vi "Curtin1_Lists.vi"(10 "Old Files":T1[](array[typedef])) -> (2 "New Files":T1[](array[typedef]))   [LabVIEW 2022 SP3]
uses:
  Curtin1_Label.ctl
panel:
  in  "Append":bool
  in  "description":string
  in  "Replace":bool
  in  "Add List":bool
  in  "Save As":bool
  in  "Save":bool
  in  "delete":bool
  in  "Export":bool
  in  "Remove":bool
  in  "List Files":i32[](listbox)
  in  "Add":bool
  in  "Possible Lists":i32(listbox)
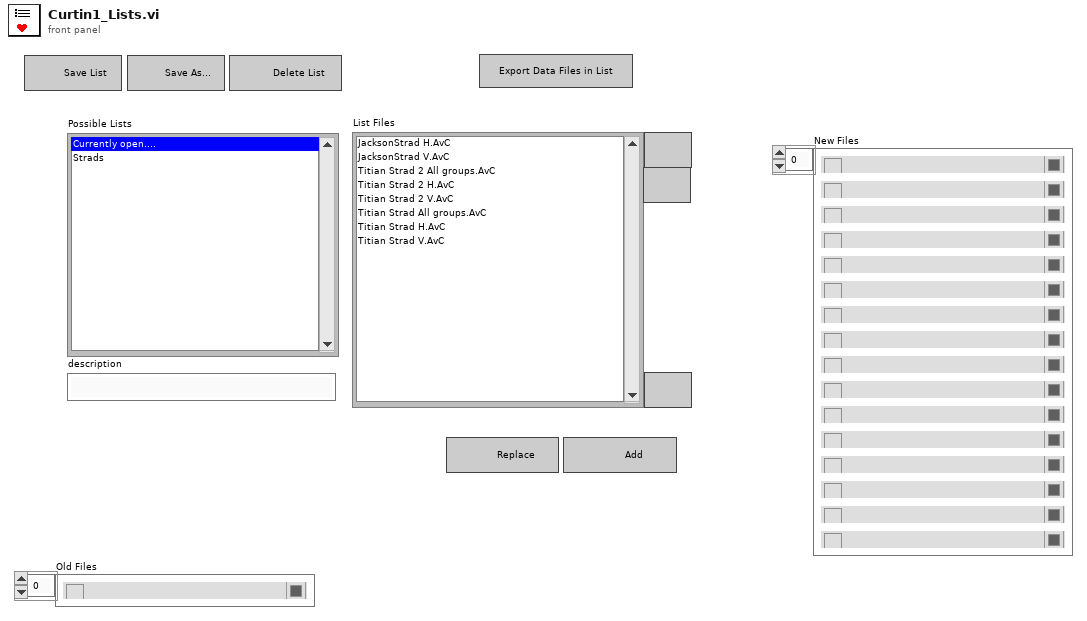
[diagram p1: front panel]
types:
  T1 = typedef "Curtin1_Label.ctl" = cluster{"Show?":bool, "Name":string, "Color":u32, "Path":path, "Show Notes":bool}
  T2 = enum8{"Enabled", "Disabled", "Disabled and Grayed Out"}
  T3 = enum32{"Invalid", "Default", "Floating", "Floating/Auto-Hide", "Modal"}
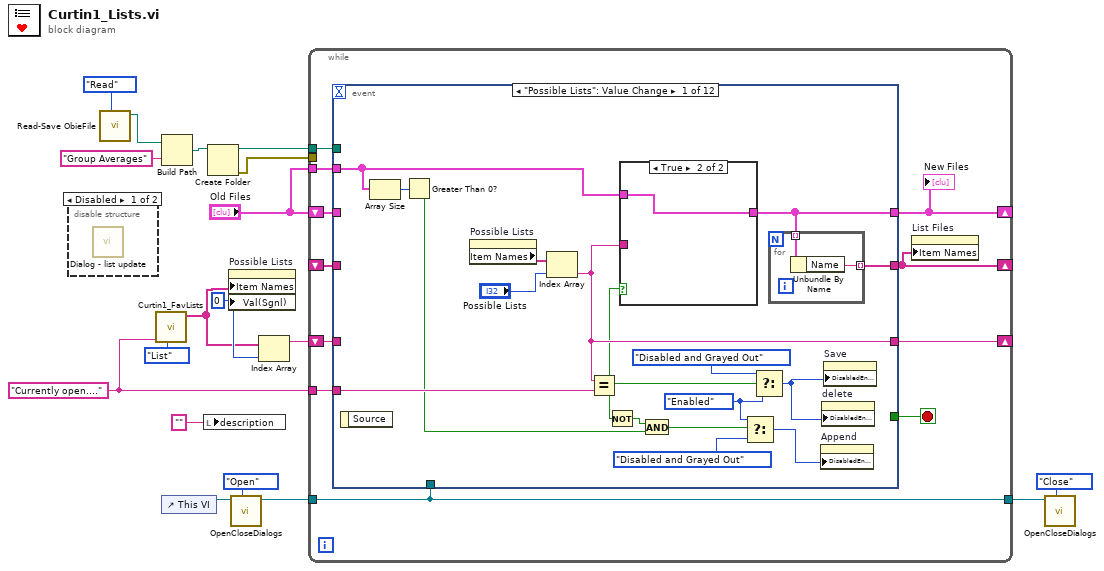
[diagram p0: block diagram]
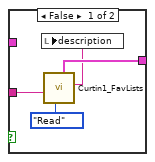
[diagram p3: hidden frame]
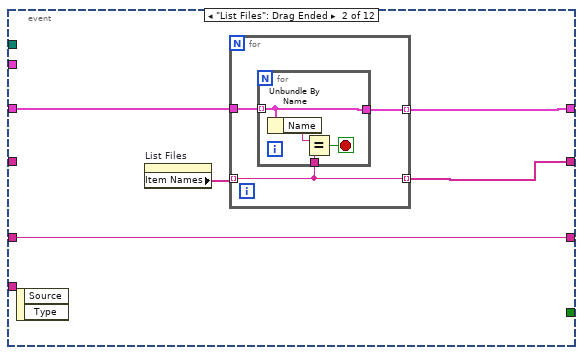
[diagram p4: hidden frame]
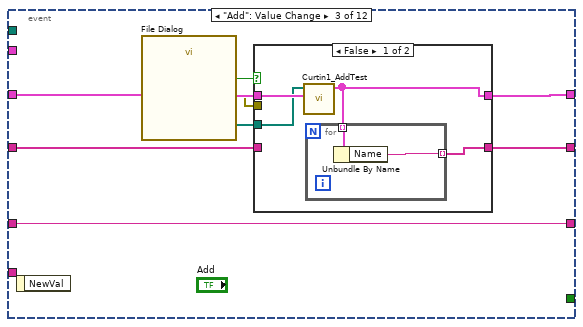
[diagram p5: hidden frame]
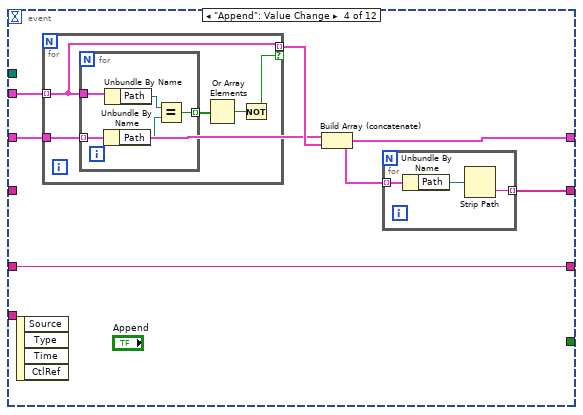
[diagram p7: hidden frame]
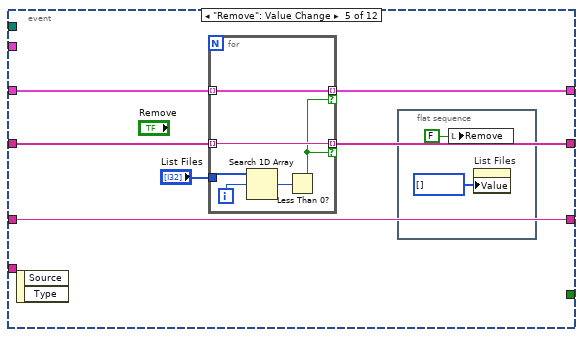
[diagram p8: hidden frame]
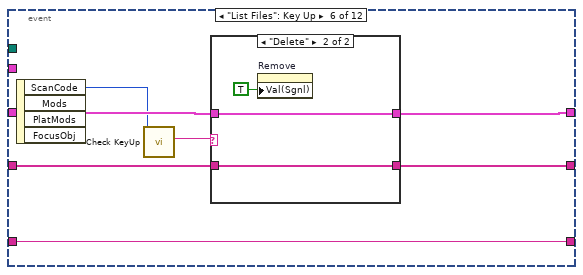
[diagram p9: hidden frame]
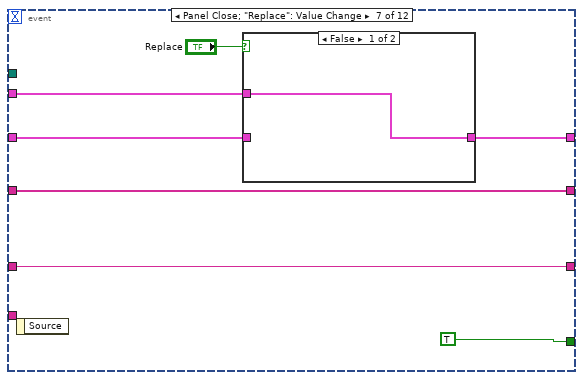
[diagram p11: hidden frame]
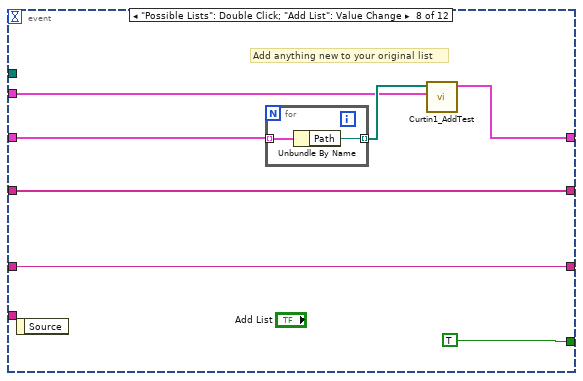
[diagram p13: hidden frame]
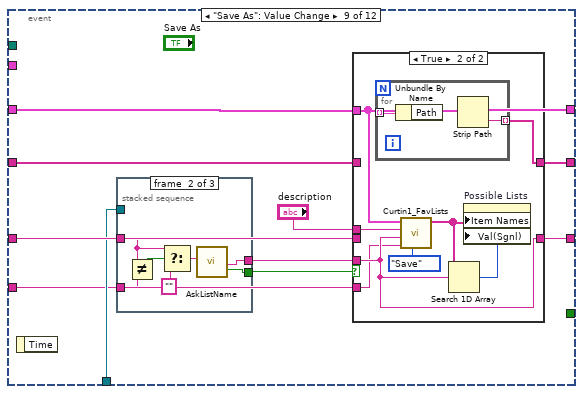
[diagram p14: hidden frame]
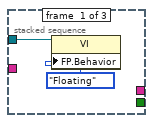
[diagram p15: hidden frame]
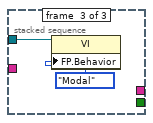
[diagram p16: hidden frame]
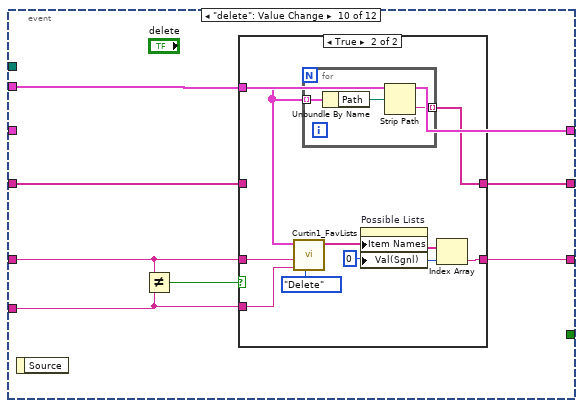
[diagram p18: hidden frame]
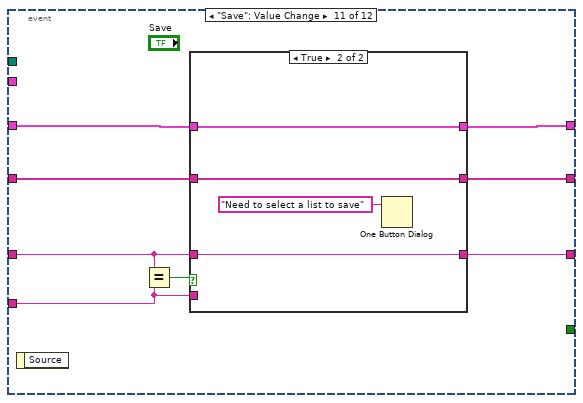
[diagram p20: hidden frame]
diagram:
  w14 = "Currently open...." ("List Name")
  w18 = u16 0 ("Value (Signaling)")
  n1 = disable-structure shown="Disabled" {
    frame Disabled {
      n2 = call "Dialog - list update.vi"() -> ()  [unwired: 10 in, 2 out]
    }
    frame Enabled {
    }
  }
  n3 = call "Read-Save ObieFile.vi"("Task"=enum16{"Save", "Read"}."Read") -> ("DataPath Out"=w12:path)  [unwired: 8 in, 2 out]
  n4 = call "Curtin1_FavLists.vi"("Task"=enum16{"Save", "Read", "List"}."List", "Default"=w14) -> ("Lists"=w1:string[])  [unwired: 6 in, 3 out]
  n5 = Build Path(base path=w12, name or relative path="Group Averages") -> (appended path=w10:path)
  n6 = control-ref of="This VI"() -> (w6:refnum<vi>)
  n7 = local write "description"("" ("description")) -> ()
  n8 = Create Folder(path (use dialog)=w10) -> (created path=w9:path, error out=w8:errorcluster)  [unwired: 2 in, 1 out]
  n9 = property on="Possible Lists" class="LstBox (strict)"("Item Names"=w1, "Val(Sgnl)"=w18) -> ()  [unwired: 2 in, 2 out]
  n10 = call "OpenCloseDialogs.vi"("Task"=enum16{"Open", "Close"}."Open", "VI in"=w6) -> ("VI out"=w3:refnum<vi>)  [unwired: 8 in, 1 out]
  n11 = Index Array(array=w1, index=w18) -> (element=w17:string)
  n12 = while {
    shift-right: [w28] -> _
    shift-left: _ -> [w29]
    shift-right: [w26] -> _
    shift-left: w17 -> [w25]
    shift-right: [w20] -> _
    shift-left: "Old Files" -> [w24]
    tunnel: "Old Files" -> [w23]
    tunnel: w14 -> [w22]
    tunnel: w9 -> [w21]
    tunnel: w8 -> [_]
    tunnel: [w19] -> w4
    tunnel: w3 -> [w19]
    stop <- w27 stop-if-true
    n13 = event shown="[0] \"Possible Lists\": Value Change" {
      selector: _ -> [_ _ _ _ _ _ _ _ _ _ _ _]
      dyn-events: _ -> [_ _ _ _ _ _ _ _ _ _ _ _]
      timeout: _ -> [_ _ _ _ _ _ _ _ _ _ _ _]
      tunnel: w29 -> [_ _ w73 _ w101 w121 w132 w142 w153 w179 w200 w223]
      tunnel: [w44 w55 w72 w82 w102 w120 w132 w142 w154 w184 w201 w223] -> w28
      tunnel: [_ _ _ _ _ _ TRUE ("OK Button") TRUE ("OK Button") _ _ _ _] -> w27
      tunnel: [w41 w54 w69 w87 w106 w119 w131 w141 w152 w182 w205 w219] -> w26
      tunnel: w25 -> [_ w54 w69 w87 w106 w119 w131 w141 w150 w181 w199 w219]
      tunnel: w24 -> [_ w58 w71 w84 w103 w118 w128 w138 w151 _ w202 w222]
      tunnel: [w43 w57 w70 w83 w104 w117 w129 w137 w151 w183 w203 w222] -> w20
      tunnel: w23 -> [w38 _ _ w86 _ _ w127 w139 _ w183 _ _]
      tunnel: w22 -> [w42 _ _ _ _ _ _ _ w145 w180 w204 _]
      tunnel: w21 -> [_ _ _ _ _ _ _ _ _ _ _ _]
      tunnel: w19 -> [_ _ _ _ _ _ _ _ w147 _ _ _]
      event "Possible Lists": Value Change {
        w32 = T2."Enabled" ("Disabled")
        n14 = event-data() -> ()  [unwired: 1 in, 1 out]
        n15 = Array Size(array=w38) -> (size(s)=w37:i32)
        n16 = Greater Than 0?(x=w37) -> (x > 0?=w34:bool)
        n17 = property on="Possible Lists" class="LstBox (strict)"() -> ("Item Names"=w46:string[])  [unwired: 2 in, 2 out]
        n18 = Index Array(array=w46, index="Possible Lists") -> (element=w41:string)
        n19 = Equal?(x=w41, y=w42) -> (x = y?=w36:bool)
        n20 = Not(x=w36) -> (.not. x?=w35:bool)
        n21 = case shown="True" w36 {
          tunnel: w41 -> [w50 _]
          tunnel: [w48 w51] -> w43
          tunnel: w38 -> [_ w51]
          frame False {
            n22 = call "Curtin1_FavLists.vi"("Task"=enum16{"Save", "Read"}."Read", "List Name"=w50) -> ("description out"=w47:string, "Files Out"=w48:T1[])  [unwired: 6 in, 2 out]
            n23 = local write "description"(w47) -> ()
          }
          frame True {
          }
        }
        n24 = And(x=w35, y=w34) -> (x .and. y?=w33:bool)
        n25 = Select(t=w32, s=w33, f=T2."Disabled and Grayed Out" ("Disabled")) -> (s? t:f=w30:T2)
        n26 = Select(t=T2."Disabled and Grayed Out" ("Disabled"), s=w36, f=w32) -> (s? t:f=w39:T2)
        n27 = for {
          tunnel: [w53] -> w44 mode=indexing
          tunnel: w43 -> [w52] mode=indexing
          n28 = Unbundle By Name(w52) -> ("Name"=w53:string)
        }
        n29 = property on="Append" class="Bool"("DisabledEnum"=w30) -> ()  [unwired: 2 in, 2 out]
        n30 = property on="delete" class="Bool"("DisabledEnum"=w39) -> ()  [unwired: 2 in, 2 out]
        n31 = property on="Save" class="Bool"("DisabledEnum"=w39) -> ()  [unwired: 2 in, 2 out]
      }
      event "List Files": Drag Ended {
        n32 = event-data() -> ()  [unwired: 1 in, 2 out]
        n33 = property on="List Files" class="LstBox (strict)"() -> ("Item Names"=w56:string[])  [unwired: 2 in, 2 out]
        n34 = for {
          tunnel: w58 -> [w61]
          tunnel: w56 -> [w59] mode=indexing
          tunnel: [w60] -> w57 mode=indexing
          tunnel: [w59] -> w55 mode=indexing
          n35 = for {
            tunnel: w61 -> [w62] mode=indexing
            tunnel: w59 -> [w64]
            tunnel: [w62] -> w60
            stop <- w63 stop-if-true
            n36 = Unbundle By Name(w62) -> ("Name"=w65:string)
            n37 = Equal?(x=w65, y=w64) -> (x = y?=w63:bool)
          }
        }
      }
      event "Add": Value Change {
        n38 = event-data() -> ()  [unwired: 1 in, 1 out]
        n39 = call "File Dialog"() -> ("selected paths"=w66:path[], "cancelled"=w68:bool, "error out"=w67:errorcluster)  [unwired: 12 in, 1 out]
        n40 = case shown="False" w68 {
          tunnel: w66 -> [w76 _]
          tunnel: w73 -> [_ w81]
          tunnel: [w74 w81] -> w72
          tunnel: w67 -> [_ _]
          tunnel: w71 -> [w77 w80]
          tunnel: [w75 w80] -> w70
          frame False {
            n41 = call "Curtin1_AddTest.vi"("Old Files"=w77, "Selected Paths"=w76) -> ("New Files"=w75:T1[])  [unwired: 9 in]
            n42 = for {
              tunnel: w75 -> [w79] mode=indexing
              tunnel: [w78] -> w74 mode=indexing
              n43 = Unbundle By Name(w79) -> ("Name"=w78:string)
            }
          }
          frame True {
          }
        }
      }
      event "Append": Value Change {
        n44 = event-data() -> ()  [unwired: 1 in, 4 out]
        n45 = for {
          tunnel: w84 -> [w93]
          tunnel: w86 -> [w92] mode=indexing
          tunnel: [w92] -> w85 mode=indexing if=w91
          n46 = for {
            tunnel: w93 -> [w100] mode=indexing
            tunnel: w92 -> [w99]
            tunnel: [w96] -> w95 mode=indexing
            n47 = Unbundle By Name(w100) -> ("Path"=w97:path)
            n48 = Unbundle By Name(w99) -> ("Path"=w98:path)
            n49 = Equal?(x=w98, y=w97) -> (x = y?=w96:bool)
          }
          n50 = Or Array Elements(Boolean array=w95) -> (logical OR=w94:bool)
          n51 = Not(x=w94) -> (.not. x?=w91:bool)
        }
        n52 = Build Array (concatenate)(w84, w85) -> (w83:T1[])
        n53 = for {
          tunnel: w83 -> [w90] mode=indexing
          tunnel: [w89] -> w82 mode=indexing
          n54 = Unbundle By Name(w90) -> ("Path"=w88:path)
          n55 = Strip Path(path=w88) -> (name=w89:string)  [unwired: 1 out]
        }
      }
      event "Remove": Value Change {
        n56 = event-data() -> ()  [unwired: 1 in, 2 out]
        n57 = for {
          tunnel: "List Files" -> [w111]
          tunnel: [w114] -> w104 mode=indexing if=w109
          tunnel: w103 -> [w114] mode=indexing
          tunnel: [w113] -> w102 mode=indexing if=w109
          tunnel: w101 -> [w113] mode=indexing
          i -> [w112]
          n58 = Search 1D Array(1D array=w111, element=w112) -> (index of element=w110:i32)  [unwired: 1 in]
          n59 = Less Than 0?(x=w110) -> (x < 0?=w109:bool)
        }
        n60 = flat-sequence {
          frame #0 {
            n61 = local write "Remove"(FALSE ("Remove")) -> ()
            n62 = property on="List Files" class="LstBox (strict)"("Value"=i32[] [] ("List Files")) -> ()  [unwired: 2 in, 2 out]
          }
        }
      }
      event "List Files": Key Up {
        n63 = event-data() -> ("ScanCode"=w115:i16)  [unwired: 1 in, 3 out]
        n64 = call "Check KeyUp.vi"("ScanCode"=w115) -> ("Task"=w116:string)  [unwired: 10 in]
        n65 = case shown="\"Delete\"" w116 {
          tunnel: w121 -> [w122 w125]
          tunnel: [w122 w125] -> w120
          tunnel: w118 -> [w123 w126]
          tunnel: [w123 w126] -> w117
          frame Default {
          }
          frame "Delete" {
            n66 = property on="Remove" class="Bool (strict)"("Val(Sgnl)"=TRUE ("Value (Signaling)")) -> ()  [unwired: 2 in, 2 out]
          }
        }
      }
      event Panel Close; "Replace": Value Change {
        n67 = event-data() -> ()  [unwired: 1 in, 1 out]
        n68 = case shown="False" "Replace" {
          tunnel: [w134 w135] -> w129
          tunnel: w128 -> [_ w135]
          tunnel: w127 -> [w134 _]
          frame False {
          }
          frame True {
          }
        }
      }
      event "Possible Lists": Double Click; "Add List": Value Change {
        # "Add anything new to your original list"
        n69 = event-data() -> ()  [unwired: 1 in, 1 out]
        n70 = for {
          tunnel: w138 -> [w144] mode=indexing
          tunnel: [w143] -> w140 mode=indexing
          n71 = Unbundle By Name(w144) -> ("Path"=w143:path)
        }
        n72 = call "Curtin1_AddTest.vi"("Old Files"=w139, "Selected Paths"=w140) -> ("New Files"=w137:T1[])  [unwired: 9 in]
      }
      event "Save As": Value Change {
        n73 = event-data() -> ()  [unwired: 1 in, 1 out]
        n74 = stacked-sequence {
          tunnel: w147 -> [w156 _ w165]
          tunnel: w150 -> [_ w159 _]
          tunnel: [_ w163 _] -> w149
          tunnel: [_ w162 _] -> w148
          tunnel: w145 -> [_ w161 _]
          frame #0 {
            n75 = property class="VI"(reference=w156, "FP.Behavior"=T3."Floating" ("Front Panel Window:Behavior")) -> ()  [unwired: 1 in, 2 out]
          }
          frame #1 {
            n76 = Not Equal?(x=w159, y=w161) -> (x != y?=w160:bool)
            n77 = Select(t=w159, s=w160, f="") -> (s? t:f=w158:string)
            n78 = call "AskListName.vi"("Default name"=w158) -> ("List"=w163:string, "OK"=w162:bool)  [unwired: 16 in, 1 out]
          }
          frame #2 {
            n79 = property class="VI"(reference=w165, "FP.Behavior"=T3."Modal" ("Front Panel Window:Behavior")) -> ()  [unwired: 1 in, 2 out]
          }
        }
        n80 = case shown="True" w148 {
          tunnel: w149 -> [_ w170]
          tunnel: [w167 w174] -> w154
          tunnel: w153 -> [w167 _]
          tunnel: [w166 w170] -> w152
          tunnel: w151 -> [_ w171]
          tunnel: w145 -> [_ w169]
          tunnel: w150 -> [w166 _]
          tunnel: "description" -> [_ w168]
          frame False {
          }
          frame True {
            n81 = for {
              tunnel: w171 -> [w178] mode=indexing
              tunnel: [w177] -> w174 mode=indexing
              n82 = Unbundle By Name(w178) -> ("Path"=w176:path)
              n83 = Strip Path(path=w176) -> (name=w177:string)  [unwired: 1 out]
            }
            n84 = call "Curtin1_FavLists.vi"("Task"=enum16{"Save", "Read", "List"}."Save", "Default"=w169, "List Name"=w170, "description in"=w168, "Files"=w171) -> ("Lists"=w172:string[])  [unwired: 3 in, 3 out]
            n85 = Search 1D Array(1D array=w172, element=w170) -> (index of element=w175:i32)  [unwired: 1 in]
            n86 = property on="Possible Lists" class="LstBox (strict)"("Item Names"=w172, "Val(Sgnl)"=w175) -> ()  [unwired: 2 in, 2 out]
          }
        }
      }
      event "delete": Value Change {
        n87 = event-data() -> ()  [unwired: 1 in, 1 out]
        n88 = Not Equal?(x=w181, y=w180) -> (x != y?=w185:bool)
        n89 = case shown="True" w185 {
          tunnel: w181 -> [_ w193]
          tunnel: [w186 w195] -> w184
          tunnel: [w187 w188] -> w182
          tunnel: w180 -> [w187 w191]
          tunnel: w183 -> [_ w194]
          tunnel: w179 -> [w186 _]
          frame False {
          }
          frame True {
            w189 = u16 0 ("Value (Signaling)")
            n90 = call "Curtin1_FavLists.vi"("Task"=enum16{"Save", "Read", "List", "Delete"}."Delete", "Default"=w191, "List Name"=w193, "Files"=w194) -> ("Lists"=w190:string[])  [unwired: 4 in, 3 out]
            n91 = for {
              tunnel: w194 -> [w198] mode=indexing
              tunnel: [w197] -> w195 mode=indexing
              n92 = Unbundle By Name(w198) -> ("Path"=w196:path)
              n93 = Strip Path(path=w196) -> (name=w197:string)  [unwired: 1 out]
            }
            n94 = property on="Possible Lists" class="LstBox (strict)"("Item Names"=w190, "Val(Sgnl)"=w189) -> ()  [unwired: 2 in, 2 out]
            n95 = Index Array(array=w190, index=w189) -> (element=w188:string)
          }
        }
      }
      event "Save": Value Change {
        n96 = event-data() -> ()  [unwired: 1 in, 1 out]
        n97 = Equal?(x=w199, y=w204) -> (x = y?=w206:bool)
        n98 = case shown="True" w206 {
          tunnel: [w208 w214] -> w205
          tunnel: w204 -> [w209 _]
          tunnel: [w210 w216] -> w203
          tunnel: w202 -> [w210 w216]
          tunnel: [w211 w215] -> w201
          tunnel: w200 -> [w211 w215]
          tunnel: w199 -> [w208 w214]
          frame False {
            n99 = local read "description"() -> (w207:string)
            n100 = call "Curtin1_FavLists.vi"("Task"=enum16{"Save", "Read", "List", "Delete"}."Save", "Default"=w209, "List Name"=w208, "description in"=w207, "Files"=w210) -> ()  [unwired: 3 in, 4 out]
          }
          frame True {
            n101 = One Button Dialog(message="Need to select a list to save") -> ()  [unwired: 1 in, 1 out]
          }
        }
      }
      event "Export": Value Change {
        n102 = event-data() -> ()  [unwired: 1 in, 1 out]
        n103 = call "Curtin1_GlobalFolder.vi"() -> ("LabVIEW Data Path"=w217:path)  [unwired: 1 in, 1 out]
        n104 = call "File Dialog2"("start path"=w217, "prompt"="Select a folder to place a copy of the listed instrument data files", "default name"=w219) -> ("selected path"=w221:path, "error out"=w218:errorcluster)  [unwired: 9 in, 2 out]
        n105 = case shown="No Error" w218 {
          tunnel: w222 -> [w226 _]
          tunnel: w221 -> [w225 _]
          frame No Error {
            n106 = Create Folder(path (use dialog)=w225) -> (error out=w224:errorcluster)  [unwired: 2 in, 2 out]
            n107 = case shown="No Error" w224 {
              tunnel: w226 -> [w228 _]
              tunnel: w225 -> [w227 w235]
              frame No Error {
                n108 = for {
                  tunnel: w228 -> [w233] mode=indexing
                  tunnel: w227 -> [w232]
                  n109 = Unbundle By Name(w233) -> ("Path"=w229:path)
                  n110 = Strip Path(path=w229) -> (name=w231:string)  [unwired: 1 out]
                  n111 = Build Path(base path=w232, name or relative path=w231) -> (appended path=w230:path)
                  n112 = Copy(10:w230, 11:w229) -> ()  [unwired: 3 in, 3 out]
                }
              }
              frame Error {
                n113 = Format Into String(format string="Could not create %s" ("List Name"), w235) -> (resulting string=w234:string)  [unwired: 2 in, 1 out]
                n114 = One Button Dialog(message=w234) -> ()  [unwired: 1 in, 1 out]
              }
            }
          }
          frame Error {
          }
        }
      }
    }
    "New Files" <- w20
    n115 = property on="List Files" class="LstBox (strict)"("Item Names"=w28) -> ()  [unwired: 2 in, 2 out]
  }
  n116 = call "OpenCloseDialogs.vi"("Task"=enum16{"Open", "Close"}."Close", "VI in"=w4) -> ()  [unwired: 8 in, 2 out]
